vi "Add Ships to Board.vi"(11 "Empty Board":T2[][](array[typedef])) -> (3 "My Board":T2[][](array[typedef]))   [LabVIEW 2019]
uses:
  Tile State.ctl
  Status Image.ctl
panel:
  out "Ending Position":cluster{dbl, dbl}
  out "Starting Position":cluster{dbl, dbl}
  in  "stop":bool
  out "Display":T1[][](array[typedef])
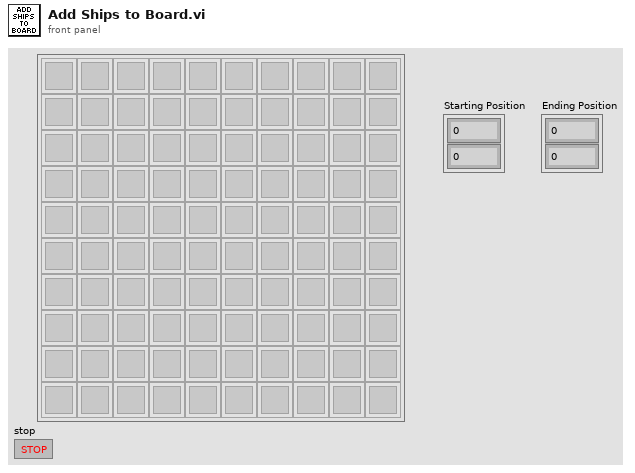
[diagram p1: front panel]
types:
  T1 = typedef "Status Image.ctl" = u16
  T2 = typedef "Tile State.ctl" = enum16{"Unknown", "Empty Water", "My Ship (Hidden)", "My Ship (Hit)", "Opponent's Ship (Revealed)", "Oponnent's Ship (Hit)"}
  T3 = typedef "LVPoint32TypeDef.ctl" = cluster{"Horizontal":i32, "Vertical":i32}
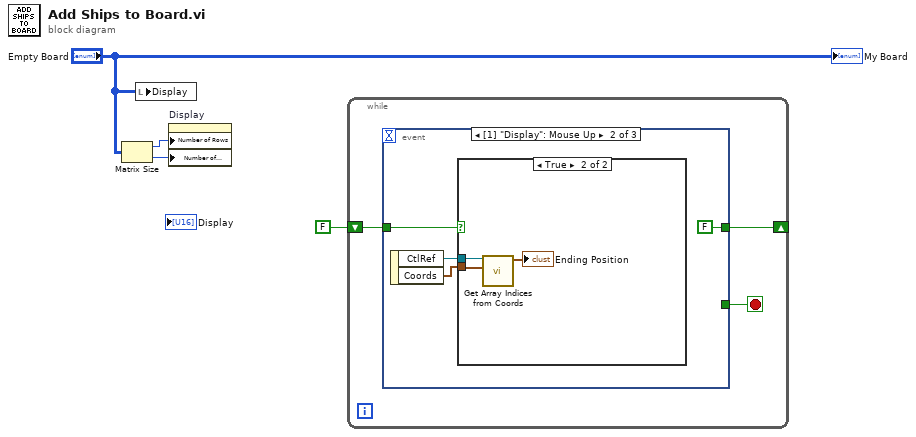
[diagram p0: block diagram]
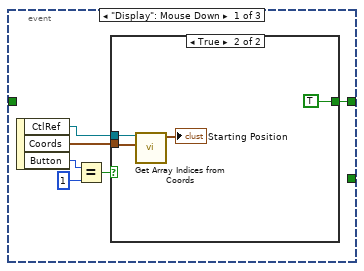
[diagram p2: hidden frame]
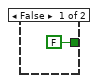
[diagram p3: hidden frame]
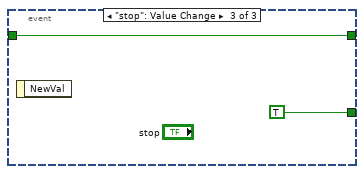
[diagram p5: hidden frame]
diagram:
  n1 = Matrix Size(0:"Empty Board") -> (1:w3:i32, 2:w4:i32)
  n2 = local write "Display"("Empty Board") -> ()
  n3 = property on="Display" class="Arr (strict)"("Number of Rows"=w3, "Number of Columns"=w4) -> ()  [unwired: 2 in, 2 out]
  n4 = while {
    shift-right: [w5] -> _
    shift-left: FALSE -> [w6]
    stop <- w7 stop-if-true
    n5 = event shown="[1] \"Display\": Mouse Up" {
      selector: _ -> [_ _ _]
      dyn-events: _ -> [_ _ _]
      timeout: _ -> [_ _ _]
      tunnel: [_ _ TRUE] -> w7
      tunnel: w6 -> [_ w19 w26]
      tunnel: [w13 FALSE ("Mouse Down") w26] -> w5
      event "Display": Mouse Down {
        n6 = event-data() -> ("CtlRef"=w8:refnum<vi>, "Coords"=w9:T3, "Button"=w12:u16)  [unwired: 1 in]
        n7 = Equal?(x=w12, y=u16 1) -> (x = y?=w10:bool)
        n8 = case shown="True" w10 {
          tunnel: [FALSE TRUE] -> w13
          tunnel: w9 -> [_ w16]
          tunnel: w8 -> [_ w17]
          frame False {
          }
          frame True {
            n9 = call "Get Array Indices from Coords.vi"("Coords"=w16, "Array in"=w17) -> ("Array Indices"=→"Starting Position":cluster{dbl, dbl})  [unwired: 9 in]
          }
        }
      }
      event "Display": Mouse Up {
        n10 = event-data() -> ("CtlRef"=w20:refnum<vi>, "Coords"=w21:T3)  [unwired: 1 in]
        n11 = case shown="True" w19 {
          tunnel: w21 -> [_ w24]
          tunnel: w20 -> [_ w25]
          frame False {
          }
          frame True {
            n12 = call "Get Array Indices from Coords.vi"("Coords"=w24, "Array in"=w25) -> ("Array Indices"=→"Ending Position":cluster{dbl, dbl})  [unwired: 9 in]
          }
        }
      }
      event "stop": Value Change {
        n13 = event-data() -> ()  [unwired: 1 in, 1 out]
      }
    }
  }
  "My Board" <- "Empty Board"
